vi "Initialize Everything Else.vi"(7 "QRD":T1, 8 "error in":errorcluster) -> (0 "error out":errorcluster, 5 "QRD Out":T1)   [LabVIEW 2025]
uses:
  Controls/Queues-Refs-Data.ctl
  Builds/Queue Wrappers.lvlibp/Q Packet.ctl
  Builds/Queue Wrappers.lvlibp
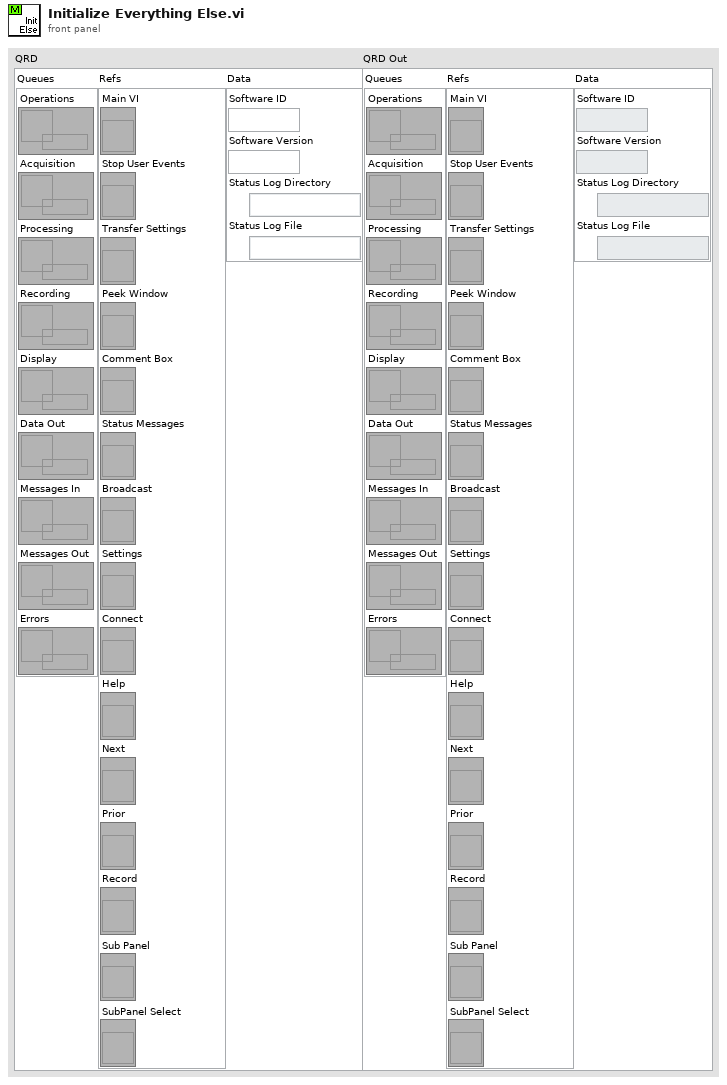
[diagram p1: front panel]
types:
  T1 = typedef "Queues-Refs-Data.ctl" = cluster{"Queues":cluster{"Operations":refnum<queue>, "Acquisition":refnum<queue>, "Processing":refnum<queue>, "Recording":refnum<queue>, "Display":refnum<queue>, "Data Out":refnum<queue>, "Messages In":refnum<queue>, "Messages Out":refnum<queue>, "Errors":refnum<queue>}, "Refs":cluster{"Main VI":refnum<vi>, "Stop User Events":refnum<vi>, "Transfer Settings":refnum<vi>, "Peek Window":refnum<vi>, "Comment Box":refnum<vi>, "Status Messages":refnum<vi>, "Broadcast":refnum<vi>, "Settings":refnum<vi>, "Connect":refnum<vi>, "Help":refnum<vi>, "Next":refnum<vi>, "Prior":refnum<vi>, "Record":refnum<vi>, "Sub Panel":refnum<vi>, "SubPanel Select":refnum<vi>}, "Data":cluster{"Software ID":string, "Software Version":string, "Status Log Directory":path, "Status Log File":path}}
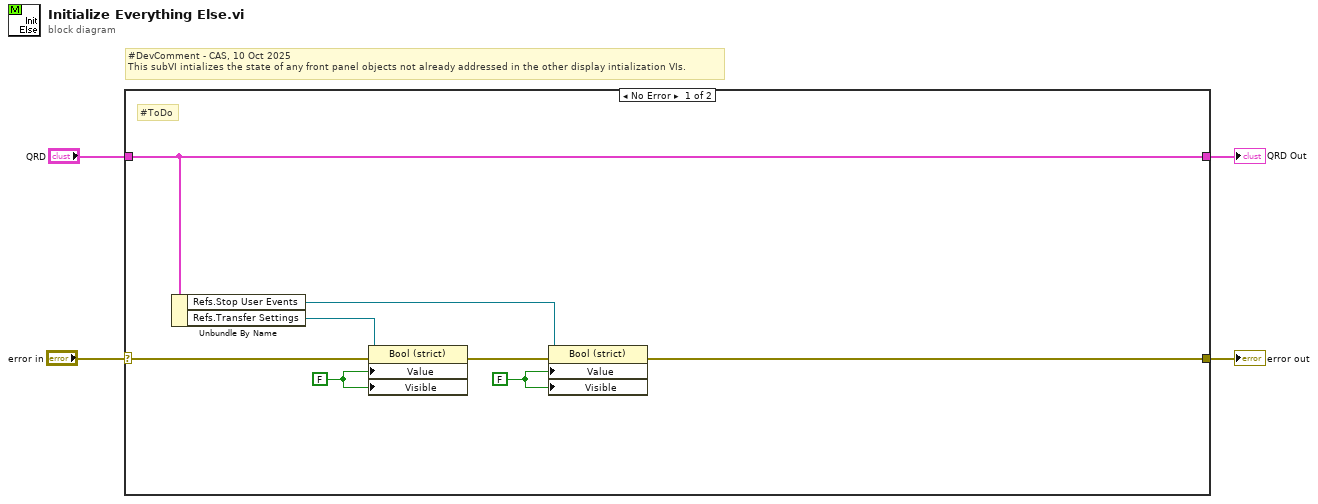
[diagram p0: block diagram]
diagram:
  # "#DevComment - CAS, 10 Oct 2025\nThis subVI intializes the state of any front panel objects not already addressed in the other display intialization VIs."
  n1 = case shown="No Error" "error in" {
    selector: "error in" -> [w8 w14]
    tunnel: "QRD" -> [w12 w13]
    tunnel: [w12 w13] -> w3
    tunnel: [w7 w14] -> w1
    frame No Error {
      w5 = FALSE ("Value")
      w6 = FALSE ("Value")
      # "#ToDo"
      n2 = Unbundle By Name(w12) -> ("Refs.Stop User Events"=w9:refnum<vi>, "Refs.Transfer Settings"=w11:refnum<vi>)
      n3 = property class="Bool (strict)"(reference=w11, error in=w8, "Value"=w6, "Visible"=w6) -> (error out=w10:errorcluster)  [unwired: 1 out]
      n4 = property class="Bool (strict)"(reference=w9, error in=w10, "Value"=w5, "Visible"=w5) -> (error out=w7:errorcluster)  [unwired: 1 out]
    }
    frame Error {
    }
  }
  "error out" <- w1
  "QRD Out" <- w3
